vi "Multiple Assert Build.vi"(8 "error in (no error)":errorcluster, 10 "GObj Array":refnum<vi>[](array[refnum]), 11 "VI in":refnum<vi>) -> (0 "error out":errorcluster)   [LabVIEW 2016]
doc: "Takes in an array of wire references to allow a user to define multiple assert vi's at once"
uses:
  Assert Build Configuration.ctl
  Core/Assert API Components/Failure Actions.ctl
  <vilib>/event_ctls.llb/eventvkey.ctl
  Numeric Operations.ctl
  String Operations.ctl
  Core/Assert API Components/Assert API Components.lvlib
panel:
  in  "Create":bool
  in  "Multiple Assert Configuration":T1[](array[typedef])
  # "Assert Name"
  # "Operation"
  # "Comparison Value (Low)"
  # "Comparison Value (High)"
  # "Comment"
  # "Default Failure Action"
  # "Description"
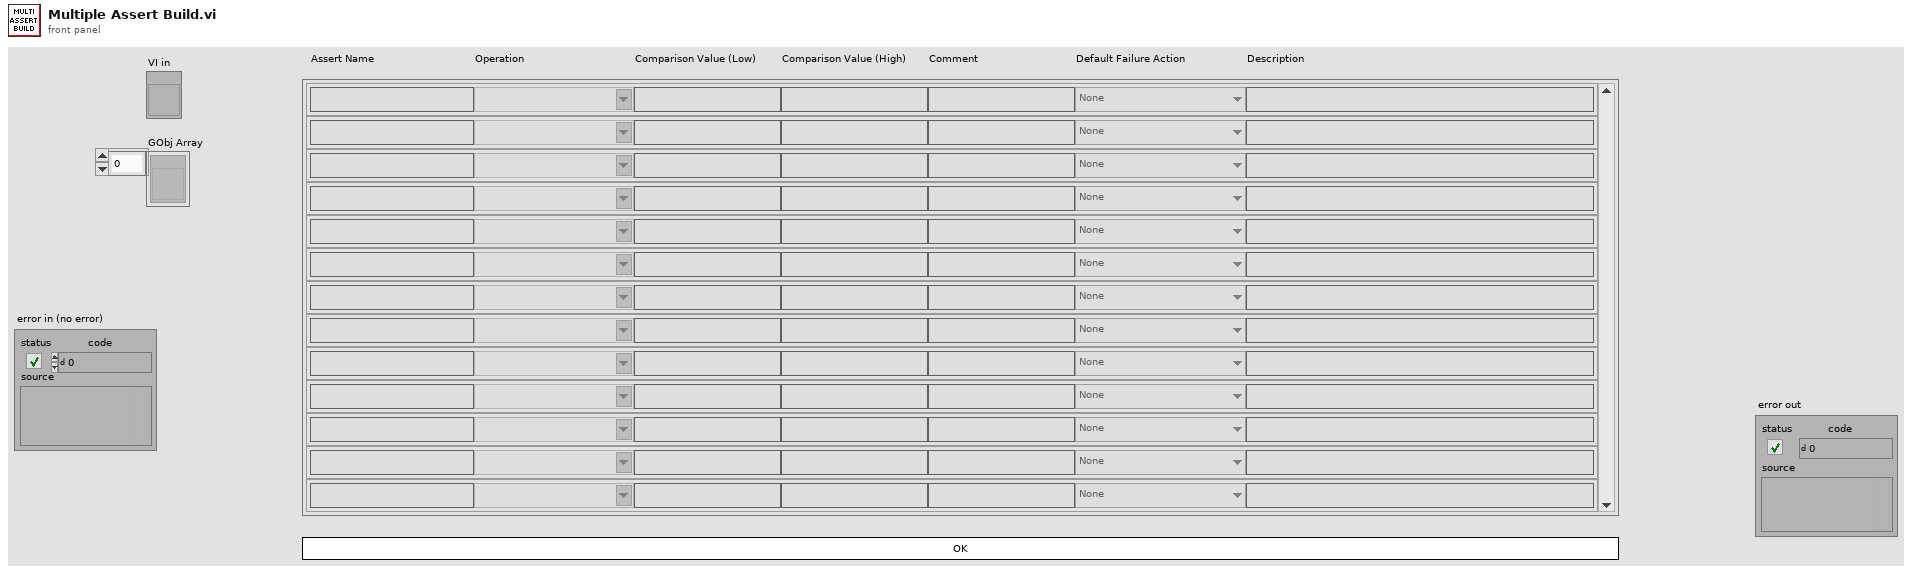
[diagram p1: front panel]
types:
  T1 = typedef "Assert Build Configuration.ctl" = cluster{"Assert Name":string, "Operation":string, "Comparison Value (Low)":string, "Comparison Value (High)":string, "Comment":string, "Default Failure Action":T2, "Description":string}
  T2 = typedef "Assert API Components.lvlib/Failure Actions.ctl" = enum16{"None", "Log To File", "Pause Execution", "Abort Execution"}
  T3 = typedef "NI_Data Type.lvlib/Data Type.ctl" = enum8{"Invalid Type", "Void", "I8", "I16", "I32", "I64", "U8", "U16", "U32", "U64", "Single Float", "Double Float", "Extended Float", "Single Complex", "Double Complex", "Extended Complex", "Enum U8", "Enum U16", "Enum U32", "Enum U64", "Single Float With Unit", "Double Float With Unit", "Extended Float With Unit", "Single Complex with Unit", "Double Complex with Unit", "Extended Complex with Unit", "Boolean", "String", "Path", "Picture", "Tag", "Array", "Cluster", "Variant", "LV Variant", "Waveform", "Timestamp", "Digital Waveform", "Digital Data", "ExpressData", "Refnum", "External Data", "VI", "Poly VI", "LabVIEW Class Instance", "Fixed Point"}
  T4 = typedef "eventvkey.ctl" = enum16{"ASCII", "Enter", "Return", "Shift", "Ctrl", "Alt", "Cmd", "Opt", "Caps", "NumLock", "Clear", "Break", "Up", "Down", "Left", "Right", "Insert", "Delete", "Home", "End", "PageUp", "PageDown", "Escape", "Help", "Pause", "ScrollLock", "F1", "F2", "F3", "F4", "F5", "F6", "F7", "F8", "F9", "F10", "F11", "F12", "F13", "F14", "F15", "F16", "F17", "F18", "F19", "F20", "F21", "F22", "F23", "F24", "Play", "VolumeUp", "VolumeDown", "Mute", "Two Byte Char"}
  T5 = typedef "Numeric Operations.ctl" = string
  T6 = typedef "String Operations.ctl" = string
  T7 = typedef "LVPoint32TypeDef.ctl" = cluster{"Horizontal":i32, "Vertical":i32}
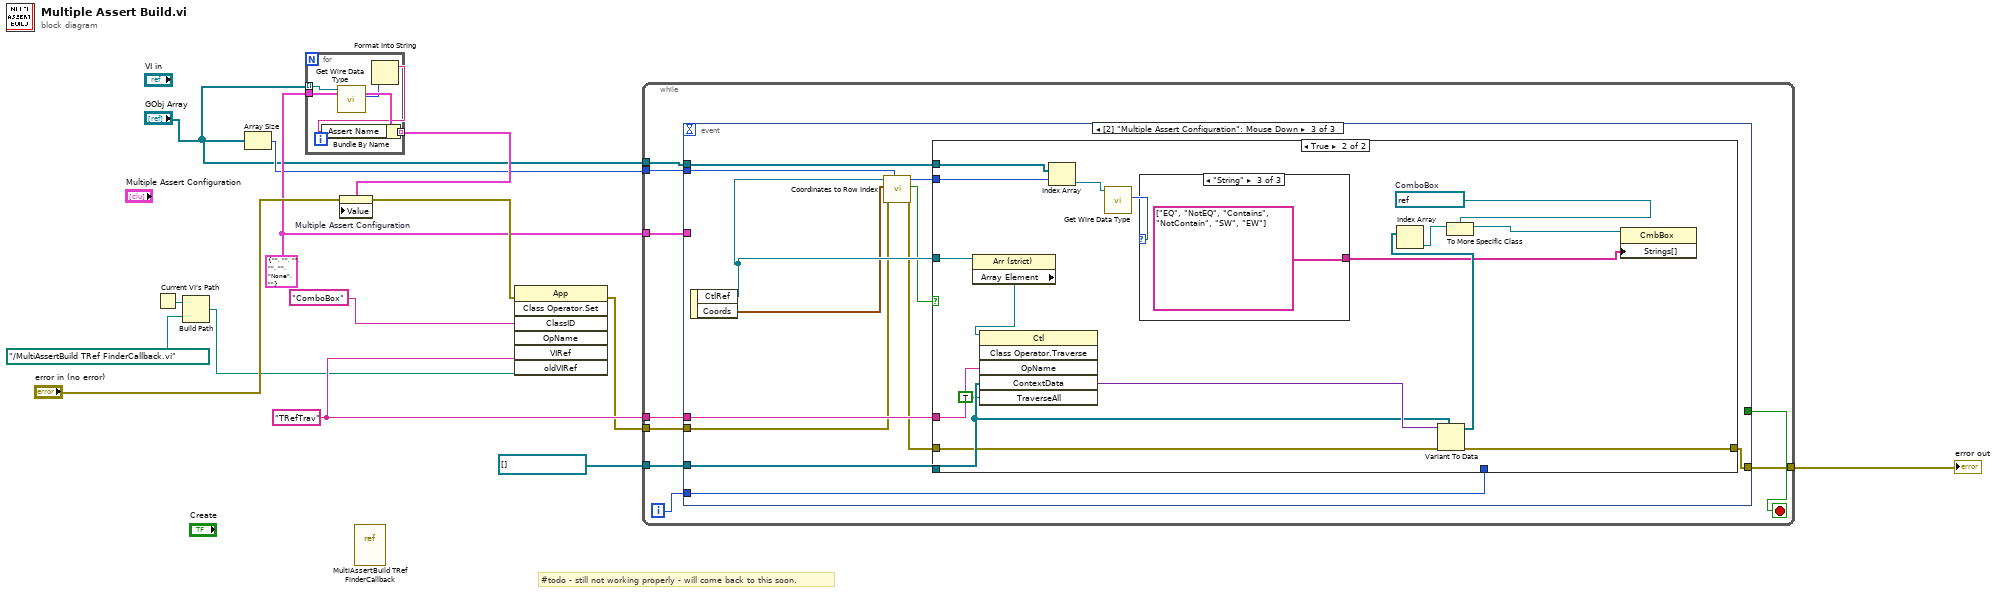
[diagram p0: block diagram]
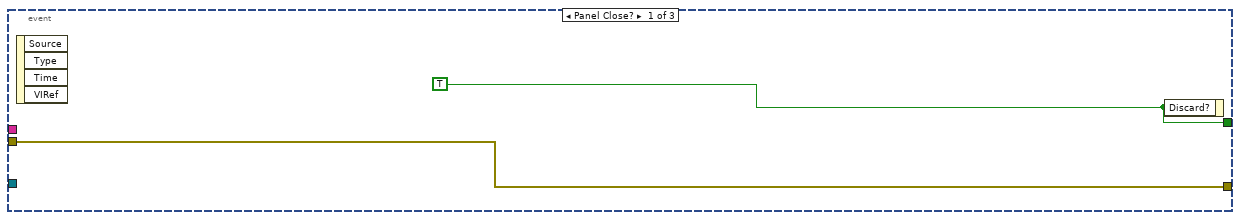
[diagram p2: hidden frame]
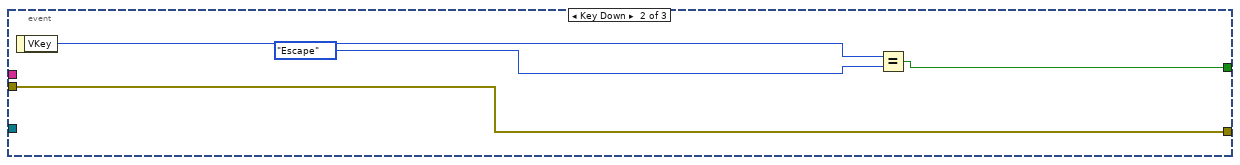
[diagram p3: hidden frame]
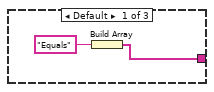
[diagram p5: hidden frame]
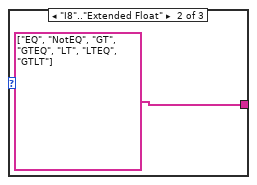
[diagram p6: hidden frame]
diagram:
  w12 = "TRefTrav"
  w3 = T1 {"Assert Name"="", "Operation"="", "Comparison Value (Low)"="", "Comparison Value (High)"="", "Comment"="", "Default Failure Action"=enum."None", "Description"=""} ("Assert Build Configuration")
  # "#todo - still not working properly - will come back to this soon."
  n1 = Current VI's Path() -> (path=w9:path)
  n2 = Build Path(base path=w9, name or relative path=path "../MultiAssertBuild TRef FinderCallback.vi" ("stripped path")) -> (appended path=w8:path)
  n3 = Array Size(array="GObj Array") -> (size(s)=w2:i32)
  n4 = for {
    tunnel: w3 -> [w18]
    tunnel: [w19] -> w4 mode=indexing
    tunnel: "GObj Array" -> [w17] mode=indexing
    n5 = call "Get Wire Data Type.vi"("Wire ref in"=w17) -> ("Type"=w16:T3)  [unwired: 8 in, 2 out]
    n6 = Format Into String(w16) -> (resulting string=w15:string)  [unwired: 3 in, 1 out]
    n7 = Bundle By Name(cluster=w18, "Assert Name"=w15) -> (w19:T1)
  }
  n8 = property on="Multiple Assert Configuration" class="Arr (strict)"(error in="error in (no error)", "Value"=w4) -> (error out=w7:errorcluster)  [unwired: 1 in, 1 out]
  n9 = vi-ref "MultiAssertBuild TRef FinderCallback.vi"() -> ()  [unwired: 1 out]
  n10 = invoke class="App" method="Class Operator.Set"(error in=w7, "ClassID"="ComboBox", "OpName"=w12, "VIRef"=w8) -> (error out=w6:errorcluster)  [unwired: 3 in, 6 out]
  n11 = while {
    tunnel: w6 -> [w27]
    tunnel: [w26] -> w13
    tunnel: w12 -> [w25]
    tunnel: refnum<vi>[] [] -> [w24]
    tunnel: w3 -> [w23]
    tunnel: w2 -> [w21]
    tunnel: "GObj Array" -> [w20]
    i -> [w22]
    stop <- w28 stop-if-true
    n12 = event shown="[2] \"Multiple Assert Configuration\": Mouse Down" {
      selector: _ -> [_ _ _]
      dyn-events: _ -> [_ _ _]
      timeout: _ -> [_ _ _]
      tunnel: [w30 w32 _] -> w28
      tunnel: w27 -> [w29 w31 w40]
      tunnel: [w29 w31 w44] -> w26
      tunnel: w25 -> [_ _ w46]
      tunnel: w24 -> [_ _ w45]
      tunnel: w23 -> [_ _ _]
      tunnel: w22 -> [_ _ w43]
      tunnel: w21 -> [_ _ w38]
      tunnel: w20 -> [_ _ w37]
      event Panel Close? {
        w30 = TRUE ("Discard?")
        n13 = event-data() -> ()  [unwired: 1 in, 4 out]
        n14 = event-data("Discard?"=w30) -> ()  [unwired: 1 in, 1 out]
      }
      event Key Down {
        n15 = event-data() -> ("VKey"=w33:T4)  [unwired: 1 in]
        n16 = Equal?(x=w33, y=eventvkey."Escape" ("VKey")) -> (x = y?=w32:bool)
      }
      event "Multiple Assert Configuration": Mouse Down {
        n17 = event-data() -> ("CtlRef"=w42:refnum<vi>, "Coords"=w41:T7)  [unwired: 1 in]
        n18 = call "Coordinates to Row Index.vi"("Number of Initalised Rows"=w38, "error in (no error)"=w40, "coords"=w41, "Array ref"=w42) -> ("error out"=w39:errorcluster, "V In Range?"=w36:bool, "row index"=w35:i16)  [unwired: 5 in]
        n19 = case shown="True" w36 {
          tunnel: w46 -> [_ w64]
          tunnel: w45 -> [_ w62]
          tunnel: [w47 w61] -> w44
          tunnel: w43 -> [_ _]
          tunnel: w42 -> [_ w58]
          tunnel: w39 -> [w47 w57]
          tunnel: w37 -> [_ w56]
          tunnel: w35 -> [_ w51]
          frame False {
          }
          frame True {
            w55 = refnum<vi> refnum  # ComboBox
            n20 = property class="Arr (strict)"(reference=w58) -> ("Array Element"=w59:refnum<vi>)  [unwired: 1 in, 2 out]
            n21 = invoke class="Ctl" method="Class Operator.Traverse"(reference=w59, "OpName"=w64, "ContextData"=w62, "TraverseAll"=TRUE ("Traverse All")) -> ("ContextData"=w63:variant)  [unwired: 2 in, 5 out]
            n22 = Index Array(array=w56, index=w51) -> (element=w50:refnum<vi>)
            n23 = call "Get Wire Data Type.vi"("Wire ref in"=w50) -> ("Type"=w49:T3)  [unwired: 8 in, 2 out]
            n24 = case shown="\"String\"" w49 {
              tunnel: [w65 T5[] ["EQ", "NotEQ", "GT", "GTEQ", "LT", "LTEQ", "GTLT"] ("Array") T6[] ["EQ", "NotEQ", "Contains", "NotContain", "SW", "EW"] ("Array")] -> w48
              frame Default {
                n25 = Build Array("Equals") -> (w65:string[])
              }
              frame "I8".."Extended Float" {
              }
              frame "String" {
              }
            }
            n26 = Variant To Data(error in=w57, type=w62, Variant=w63) -> (data=w53:refnum<vi>[], error out=w61:errorcluster)
            n27 = Index Array(array=w53) -> (element=w52:refnum<vi>)  [unwired: 1 in]
            n28 = To More Specific Class(target class=w55, reference=w52) -> (specific class reference=w54:refnum<vi>)  [unwired: 1 in, 1 out]
            n29 = property class="CmbBox"(reference=w54, "Strings[]"=w48) -> ()  [unwired: 1 in, 2 out]
          }
        }
      }
    }
  }
  "error out" <- w13
